vi "Read Current tour.vi"(8 "error in (no error)":errorcluster, 11 "Tiger Woods in":refnum<class "Tiger Woods.lvclass">) -> (0 "error out":errorcluster, 2 "Current tour":string, 3 "Tiger Woods out":refnum<class "Tiger Woods.lvclass">)   [LabVIEW 2019, in "Tiger Woods.lvclass"]
uses:
  Tiger Woods.lvclass
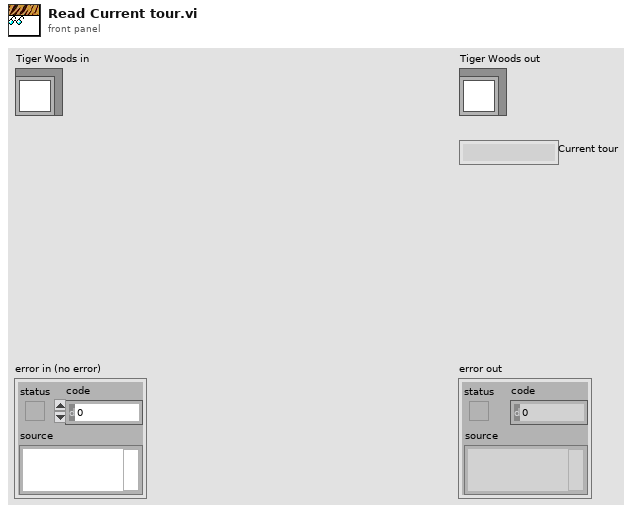
[diagram p1: front panel]
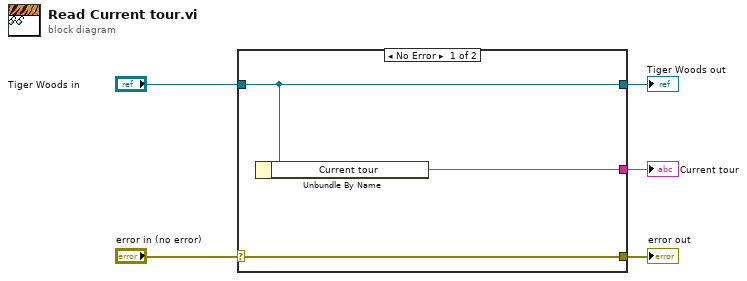
[diagram p0: block diagram]
diagram:
  n1 = case shown="No Error" "error in (no error)" {
    selector: "error in (no error)" -> [w8 w9]
    tunnel: [w8 w9] -> w4
    tunnel: [w7 w10] -> w2
    tunnel: "Tiger Woods in" -> [w7 w10]
    tunnel: [w6 _] -> w1
    frame No Error {
      n2 = Unbundle By Name(w7) -> ("Current tour"=w6:string)
    }
    frame Error {
    }
  }
  "error out" <- w4
  "Tiger Woods out" <- w2
  "Current tour" <- w1
